vi "Actor Core.vi"(8 "error in":errorcluster, 11 "Capillary in":refnum<class "Capillary.lvclass">) -> (0 "error out":errorcluster, 3 "Actor out":refnum<class "Actor.lvclass">)   [LabVIEW 2015, in "AMS UI.lvlib" / "Capillary.lvclass"]
doc: "(<B>Filename</B>: Actor Framework.lvlib:Actor.lvclass:Actor Core.vi)\n\nReceives messages to the actor, reacts to them, and initiates any error handling that may shut the actor down.\n\nDescendant classes may override this VI to append parallel tasks for the actor to complete while it handles messages. Overrides use the Call Parent Method node."
uses:
  Capillary.lvclass
  <vilib>/ActorFramework/Actor/Actor.lvclass
  <vilib>/ActorFramework/Message Enqueuer/Message Enqueuer.lvclass/Message Enqueuer.ctl
  <vilib>/ActorFramework/Message Enqueuer/Enqueue.vi
  <vilib>/ActorFramework/Message Priority Queue/Priority Enqueue.vi
  AMS Gas Actor/AMS Gas Actor.lvclass
  Capillary Messages/Indicate Capillary Line Msg/Indicate Capillary Line Msg.lvclass
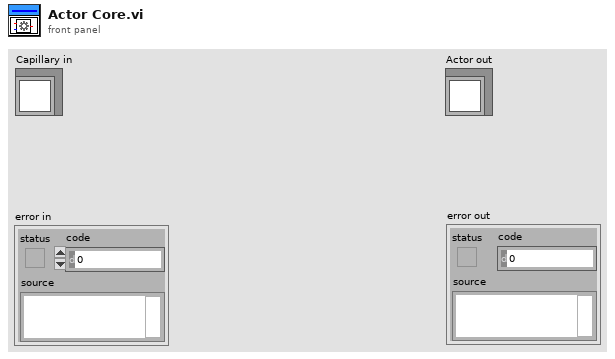
[diagram p1: front panel]
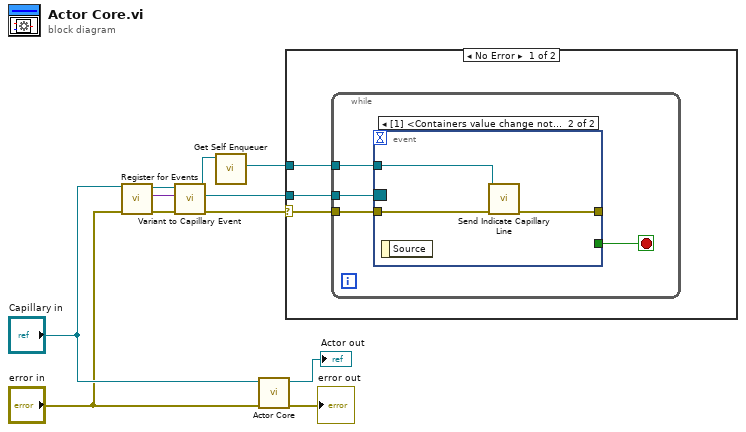
[diagram p0: block diagram]
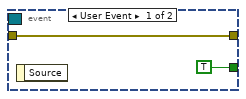
[diagram p2: hidden frame]
diagram:
  n1 = call-dynamic "Register for Events.vi"("error in (no error)"="error in", "Capillary in"="Capillary in") -> ("error out"=w7:errorcluster, "Event Registration Refnum"=w5:variant, "Capillary out"=w6:refnum<class "Capillary.lvclass">)  [unwired: 7 in]
  n2 = call "Variant to Capillary Event.vi"("error in (no error)"=w7, "variant"=w5, "Capillary in"=w6) -> ("error out"=w3:errorcluster, "Event Registration Refnum"=w1:refnum<event-registration>, "Capillary out"=w4:refnum<class "Capillary.lvclass">)  [unwired: 6 in]
  n3 = call-dynamic "Get Self Enqueuer.vi"("eActor in"=w4) -> ("Actor Framework:Message Enqueuer"=w2:refnum<class "Message Enqueuer.lvclass">)  [unwired: 9 in, 1 out]
  n4 = call-parent "Actor Core.vi"("error in"="error in", "Actor in"="Capillary in") -> ("error out"=→"error out":errorcluster, "Actor out"=→"Actor out":refnum<class "Actor.lvclass">)  [unwired: 8 in]
  n5 = case shown="No Error" w3 {
    selector: w3 -> [w13 _]
    tunnel: w1 -> [w14 _]
    tunnel: w2 -> [w12 _]
    frame No Error {
      n6 = while {
        tunnel: w14 -> [w18]
        tunnel: w13 -> [w17]
        tunnel: w12 -> [w15]
        stop <- w16 stop-if-true
        n7 = event shown="[1] <Containers value change notification>: User Event" {
          selector: w18 -> [_ _]
          dyn-events: _ -> [_ _]
          timeout: _ -> [_ _]
          tunnel: w17 -> [w19 w23]
          tunnel: [w19 w22] -> _
          tunnel: [TRUE _] -> w16
          tunnel: w15 -> [_ w21]
          event User Event {
            n8 = event-data() -> ()  [unwired: 1 in, 1 out]
          }
          event User Event {
            n9 = event-data() -> ()  [unwired: 1 in, 1 out]
            n10 = call "Send Indicate Capillary Line.vi"("error in (no error)"=w23, "Message Enqueuer"=w21) -> ("error out"=w22:errorcluster)  [unwired: 8 in, 1 out]
          }
        }
      }
    }
    frame Error {
    }
  }
